vi "axis_scan.vi"(4 "Calibration":bool, 5 "Modes":bool, 6 "Parameters":bool, 7 "Parameters in":T1={"Stimulus"={"Type"=enum."Off", "Phase"=0.0, "Amplitude"=[], "Injection point"=enum."Total pose", "Closed loop"=FALSE, "Offset"=[], "Tip -> world"=FALSE, "Frequency"=0.0, "Length"=0.0}, "Goal Filter A"={"Speedup max"=0.0, "Speedup thresh"=0.0, "Speedup nonlin"=0.0, "Filters"=[]}, "Mode controls"={"Hold"=FALSE, "Cancellation"=FALSE, "Goal filter"=FALSE, "Trigger"=FALSE}, "Manipulator type"=enum."Current piezo", "Manipulator calibration"={"Tool offsets"=[], "Tip light calibration"=[], "Handle light calibration"=[], "Base pivots"=[], "Output pivots"=[], "Length center"=0.0, "Workspace height"=[], "Workspace diameter"=[0.0, 0.0, 36200.0], "Linearization"=[], "Stack travel"=400.0, "Saturation pos"=375.0, "Inverse filters"=[]}, "Network"={"Remote Host"="", "Send Status"=FALSE, "Send Port"=0, "Recv Commands"=FALSE, "Recv Port"=0}, "Goal Filter B"={"Speedup max"=0.0, "Speedup thresh"=0.0, "Speedup nonlin"=0.0, "Filters"=[]}, "Cancellation"={"KP"={"XY"=0.0, "Rxy"=0.0, "Z"=0.0, "Rz"=0.0}, "KI"=0.0, "KD"={"XY"=0.0, "Rxy"=0.0, "Z"=0.0, "Rz"=0.0}, "Max vel"=20.0, "Max acc"=0.001, "Int error limit"=3.0, "RCM gain"=0.0, "Bypass"=FALSE, "Degraded gain"=0.0}, "Transition time"=0.0, "Estimation"={"Link"={"Measure noise"=[], "Process noise"=[], "Alt process noise"=[], "Alt turnoff cycles"=20, "Innovation limit"=[], "Residue threshold"=0.0, "Enable"=FALSE}, "Handle"={"Measure noise"=[], "Process noise"=[], "State limits"=[], "Innovation limit"=[], "Prediction Lookahead"=0.0, "Enable"=FALSE}}} {"Transition time" format="%_3f"; "Cancellation"."Degraded gain" min=0 max=1 step=0.1 format="%#_3p"; "Cancellation"."RCM gain" min=0 max=1 step=0.1 format="%#_3p"; "Cancellation"."KD"."Rz" min=0 max=1 step=0.1 format="%#_3p"; "Cancellation"."KD"."Rxy" min=0 max=1 step=0.1 format="%#_3p"; "Cancellation"."KD"."Z" min=0 max=1 step=0.1 format="%#_3p"; "Cancellation"."KD"."XY" min=0 max=1 step=0.1 format="%#_3p"; "Cancellation"."KI" min=0 max=1 step=0.01 format="%#_3p"; "Cancellation"."KP"."Rz" min=0 max=1 step=0.1 format="%#_3p"; "Cancellation"."KP"."Rxy" min=0 max=1 step=0.1 format="%#_3p"; "Cancellation"."KP"."Z" min=0 max=1 step=0.1 format="%#_3p"; "Cancellation"."KP"."XY" min=0 max=1 step=0.1 format="%#_3p"; "Cancellation"."Max acc" format="%#_3p"; "Goal Filter B"."Filters"."V limit range" format="%_3p"; "Goal Filter B"."Filters"."V limit" format="%_3p"; "Goal Filter B"."Filters"."Upper Q" format="%_3f"; "Goal Filter B"."Filters"."Upper Fc" format="%_3p"; "Goal Filter B"."Filters"."Lower Q" format="%_3f"; "Goal Filter B"."Filters"."Scale factor" format="%_3f"; "Goal Filter B"."Filters"."Lower Fc" format="%_3p"; "Goal Filter B"."Speedup nonlin" format="%_3p"; "Goal Filter B"."Speedup thresh" format="%_3p"; "Goal Filter B"."Speedup max" format="%_3p"; "Manipulator calibration"."Saturation pos" format="%#.1f"; "Manipulator calibration"."Stack travel" format="%#.1f"; "Manipulator calibration"."Output pivots" format="%#_6f"; "Manipulator calibration"."Base pivots" format="%#_6f"; "Manipulator calibration"."Handle light calibration" format="%#.1f"; "Manipulator calibration"."Tip light calibration" format="%#.1f"; "Goal Filter A"."Filters"."V limit range" format="%_3p"; "Goal Filter A"."Filters"."V limit" format="%_3p"; "Goal Filter A"."Filters"."Upper Q" format="%_3f"; "Goal Filter A"."Filters"."Upper Fc" format="%_3p"; "Goal Filter A"."Filters"."Lower Q" format="%_3f"; "Goal Filter A"."Filters"."Scale factor" format="%_3f"; "Goal Filter A"."Filters"."Lower Fc" format="%_3p"; "Goal Filter A"."Speedup nonlin" format="%_3p"; "Goal Filter A"."Speedup thresh" format="%_3p"; "Goal Filter A"."Speedup max" format="%_3p"; "Stimulus"."Length" min=0.0 max=100.0 step=100.0 format="%#_4p"; "Stimulus"."Frequency" min=0.0 step=100.0 format="%#_4g"; "Stimulus"."Offset" format="%#_3p"; "Stimulus"."Amplitude" format="%#_3p"; "Stimulus"."Phase" min=-180.0 max=360.0 step=100.0 format="%#.2f"}, 8 "Next scan occurrence":refnum<k4>, 9 "Use Output Enable":bool, 10 "Amplitude":sgl, 11 "Scan axes":bool[](array[boolean])=[FALSE, FALSE, FALSE, FALSE, FALSE, FALSE]) -> (3 "Got all":bool)   [LabVIEW 2013]
uses:
  testing/Micron params.ctl
  testing/stimulus.ctl
  testing/injection_point.ctl
  filtering/goal_loop_parms.ctl
  testing/mode_conrols.ctl
  testing/manipulator_cal.ctl
  asap/labview/testing/probe_calibration.ctl
  host/network_params.ctl
  cancellation/sq_control_params.ctl
  cancellation/decoupled_gain.ctl
  cancellation/estimation_controls.ctl
  initialization/micron_globals.vi
panel:
  # "Sequence a scan across axes by altering the stimulus amplitude.  If the injection point is in link-length coordinates and \"Use Output Enable\" is true, we also use \"output_enable\" to shut off the other axes.  \n\nThis VI does not return until the entire scan is done.  After starting each trace cycle, we wait for \"Next scan occurrence\" before going on to the next.  This occurrence should be set by the caller when they are done processing the results.  Calls ui_override to control Micron triggering and stimulus.  Additional overrides can be specified by the boolean flags, as for ui_override.   If override is not successful, then we do nothing, and \"Got all\" is false.  Information on the axis currently being driven in stored in the \"Axis scan\" global."
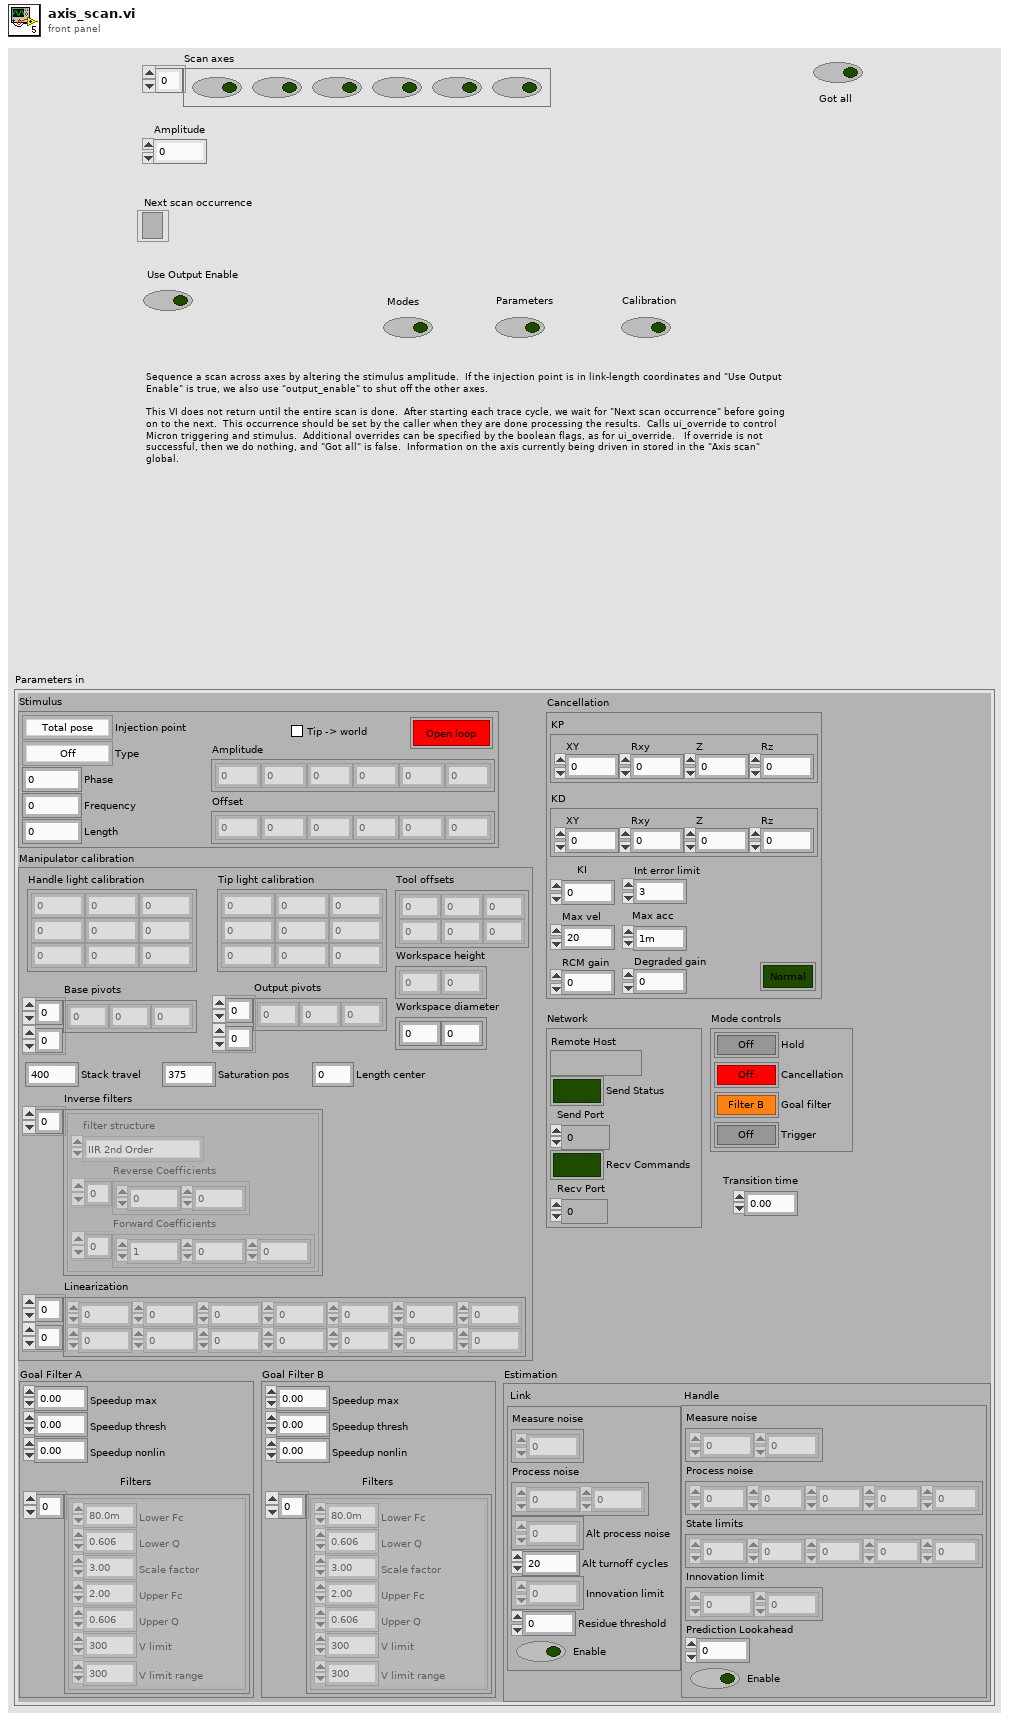
[diagram p1: front panel]
types:
  T1 = typedef "Micron params.ctl" = cluster{"Stimulus":T2, "Goal Filter A":T4, "Mode controls":T5, "Manipulator type":enum16{"Current piezo", "Voltage piezo"}, "Manipulator calibration":T6, "Network":T8, "Goal Filter B":T4, "Cancellation":T9, "Transition time":sgl, "Estimation":T11}
  T2 = typedef "stimulus.ctl" = cluster{"Type":enum16{"Off", "Step", "Sine", "Triangle", "Arbitrary"}, "Phase":dbl, "Amplitude":sgl[], "Injection point":T3, "Closed loop":bool, "Offset":sgl[], "Tip -> world":bool, "Frequency":dbl, "Length":dbl}
  T3 = typedef "injection_point.ctl" = enum16{"Total pose", "V limiter", "Goal ", "Link position", "KF link position", "Inverse kin", "Link goal", "Link error", "Controller", "Output", "Drive", "Light"}
  T4 = typedef "goal_loop_parms.ctl" = cluster{"Speedup max":sgl, "Speedup thresh":sgl, "Speedup nonlin":sgl, "Filters":cluster{"Lower Fc":sgl, "Lower Q":sgl, "Scale factor":sgl, "Upper Fc":sgl, "Upper Q":sgl, "V limit":sgl, "V limit range":sgl}[]}
  T5 = typedef "mode_conrols.ctl" = cluster{"Hold":bool, "Cancellation":bool, "Goal filter":bool, "Trigger":bool}
  T6 = typedef "manipulator_cal.ctl" = cluster{"Tool offsets":sgl[][], "Tip light calibration":T7, "Handle light calibration":T7, "Base pivots":sgl[][], "Output pivots":sgl[][], "Length center":sgl, "Workspace height":sgl[], "Workspace diameter":sgl[], "Linearization":sgl[][], "Stack travel":sgl, "Saturation pos":sgl, "Inverse filters":cluster{"filter structure":enum32{"IIR 2nd Order", "IIR 4th Order"}, "Reverse Coefficients":dbl[], "Forward Coefficients":dbl[]}[]}
  T7 = typedef "probe_calibration.ctl" = sgl[][]
  T8 = typedef "network_params.ctl" = cluster{"Remote Host":string, "Send Status":bool, "Send Port":u16, "Recv Commands":bool, "Recv Port":u16}
  T9 = typedef "sq_control_params.ctl" = cluster{"KP":T10, "KI":sgl, "KD":T10, "Max vel":sgl, "Max acc":sgl, "Int error limit":sgl, "RCM gain":sgl, "Bypass":bool, "Degraded gain":sgl}
  T10 = typedef "decoupled_gain.ctl" = cluster{"XY":sgl, "Rxy":sgl, "Z":sgl, "Rz":sgl}
  T11 = typedef "estimation_controls.ctl" = cluster{"Link":cluster{"Measure noise":dbl[], "Process noise":dbl[], "Alt process noise":dbl[], "Alt turnoff cycles":i32, "Innovation limit":dbl[], "Residue threshold":dbl, "Enable":bool}, "Handle":cluster{"Measure noise":dbl[], "Process noise":dbl[], "State limits":dbl[], "Innovation limit":dbl[], "Prediction Lookahead":sgl, "Enable":bool}}
  T12 = typedef "ui_override_opts.ctl" = cluster{"Triggering":bool, "Parameters":bool, "Stimulus":bool, "Calibration":bool, "Modes":bool}
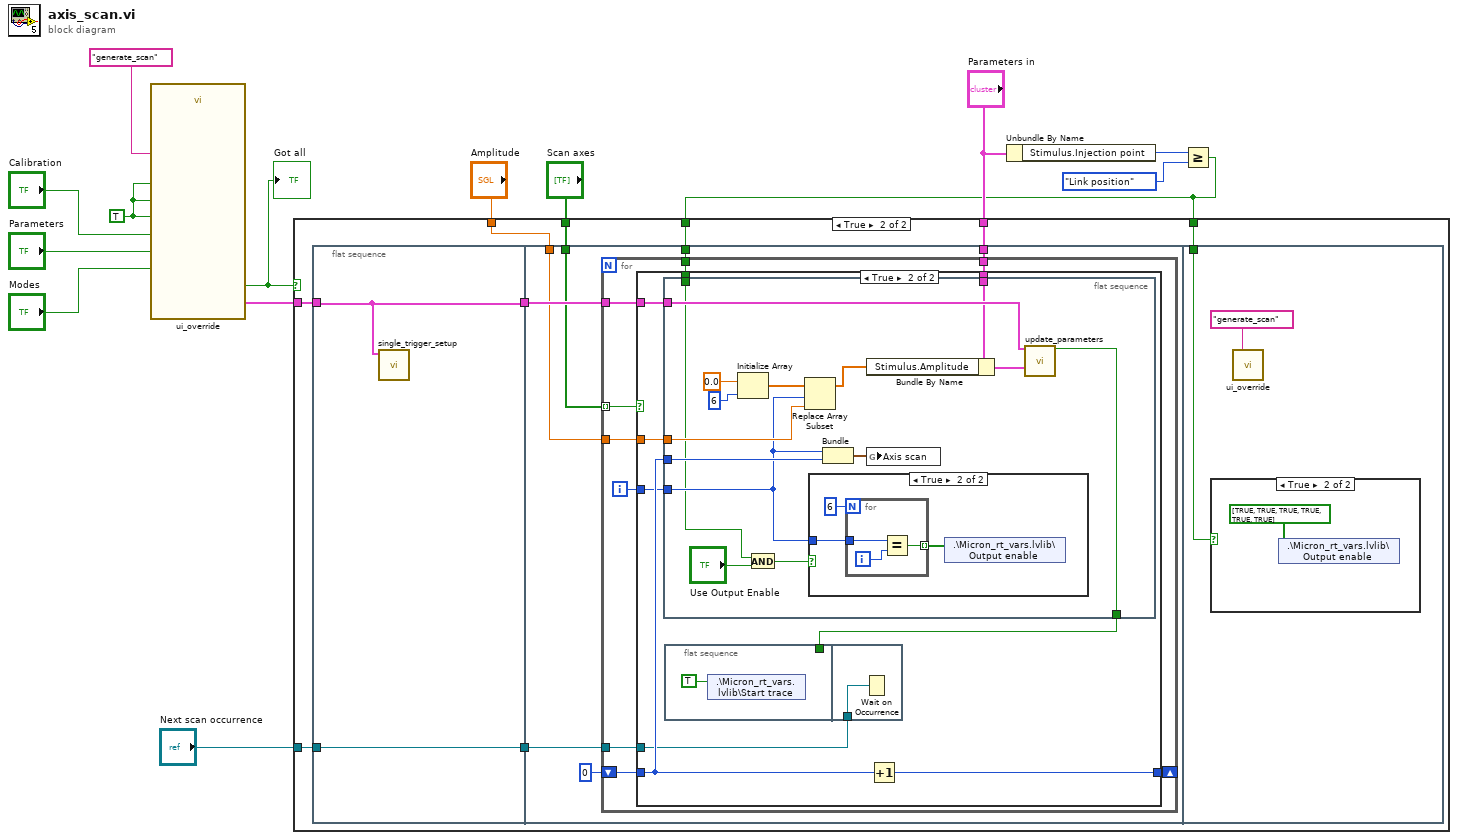
[diagram p0: block diagram]
diagram:
  w10 = TRUE ("Triggering")
  n1 = call "ui_override.vi"("Triggering"=w10, "VI name"="generate_scan", "Parameters"="Parameters", "Stimulus"=w10, "Calibration"="Calibration", "All or nothing"=w10, "Modes"="Modes") -> ("Override"=w12:T12, "Got all"=w11:bool)  [unwired: 6 in, 1 out]
  "Got all" <- w11
  n2 = Unbundle By Name("Parameters in") -> ("Stimulus.Injection point"=w3:T3)
  n3 = Greater Or Equal?(x=w3, y=injection_point."Link position") -> (x >= y?=w1:bool)
  n4 = case shown="True" w11 {
    tunnel: "Next scan occurrence" -> [_ w23]
    tunnel: w12 -> [_ w22]
    tunnel: "Parameters in" -> [_ w19]
    tunnel: "Scan axes" -> [_ w18]
    tunnel: "Amplitude" -> [_ w17]
    tunnel: w1 -> [_ w16]
    tunnel: w1 -> [_ w15]
    frame False {
    }
    frame True {
      n5 = flat-sequence {
        tunnel: w23 -> [w24]
        tunnel: [w24] -> w21
        tunnel: w22 -> [w25]
        tunnel: [w25] -> w20
        tunnel: w21 -> [w31]
        tunnel: w20 -> [w30]
        tunnel: w19 -> [w29]
        tunnel: w18 -> [w28]
        tunnel: w17 -> [w27]
        tunnel: w16 -> [w26]
        tunnel: w15 -> [w75]
        frame #0 {
          n6 = call "single_trigger_setup.vi"("Override in"=w25) -> ()  [unwired: 10 in, 1 out]
        }
        frame #1 {
          n7 = for {
            tunnel: w28 -> [w41] mode=indexing
            shift-right: [w39] -> _
            shift-left: 0 ("dimension size") -> [w40]
            tunnel: w31 -> [w38]
            tunnel: w30 -> [w36]
            tunnel: w29 -> [w35]
            tunnel: w27 -> [w34]
            tunnel: w26 -> [w33]
            i -> [w37]
            n8 = case shown="True" w41 {
              tunnel: w40 -> [w42 w50]
              tunnel: [w42 w51] -> w39
              tunnel: w38 -> [_ w48]
              tunnel: w37 -> [_ w47]
              tunnel: w36 -> [_ w46]
              tunnel: w35 -> [_ w45]
              tunnel: w34 -> [_ w44]
              tunnel: w33 -> [_ w43]
              frame False {
              }
              frame True {
                n9 = flat-sequence {
                  tunnel: w50 -> [w58]
                  tunnel: [w64] -> w49
                  tunnel: w47 -> [w57]
                  tunnel: w46 -> [w63]
                  tunnel: w45 -> [w61]
                  tunnel: w44 -> [w60]
                  tunnel: w43 -> [w55]
                  frame #0 {
                    n10 = Initialize Array(sgl 0.0 ("Amplitude"), 6 ("dimension size")) -> (w66:sgl[])
                    n11 = And(x=w55, y="Use Output Enable") -> (x .and. y?=w54:bool)
                    n12 = Replace Array Subset(array=w66, new element=w60, index=w57) -> (w65:sgl[])
                    n13 = case shown="True" w54 {
                      tunnel: w57 -> [_ w70]
                      frame False {
                      }
                      frame True {
                        n14 = for {
                          N: 6 -> [_]
                          tunnel: w70 -> [w73]
                          tunnel: [w72] -> w69 mode=indexing
                          i -> [w74]
                          n15 = Equal?(x=w73, y=w74) -> (x = y?=w72:bool)
                        }
                        n16 = shared-variable ".\\Micron_rt_vars.lvlib\\Output enable"(w69) -> ()  [unwired: 1 in, 1 out]
                      }
                    }
                    n17 = Bundle(w57, "dimension size"=w58) -> (w59:cluster{i32, "dimension size":i32})  [unwired: 1 in]
                    n18 = Bundle By Name(cluster=w61, "Stimulus.Amplitude"=w65) -> (w62:T1)
                    n19 = global write "micron_globals.vi" "Axis scan"(w59) -> ()
                    n20 = call "update_parameters.vi"("Modify"=w63, "Parameters"=w62) -> ("Changed"=w64:bool)  [unwired: 12 in, 1 out]
                  }
                }
                n21 = flat-sequence {
                  tunnel: w49 -> [_]
                  tunnel: w48 -> [w53]
                  frame #0 {
                    n22 = shared-variable ".\\Micron_rt_vars.lvlib\\Start trace"(TRUE ("Start trace")) -> ()  [unwired: 2 out]
                  }
                  frame #1 {
                    n23 = Wait on Occurrence(2:w53) -> ()  [unwired: 2 in, 1 out]
                  }
                }
                n24 = Increment(x=w50) -> (x+1=w51:i32)
              }
            }
          }
        }
        frame #2 {
          n25 = case shown="True" w75 {
            frame False {
            }
            frame True {
              n26 = shared-variable ".\\Micron_rt_vars.lvlib\\Output enable"(bool[] [TRUE, TRUE, TRUE, TRUE, TRUE, TRUE] ("Output enable")) -> ()  [unwired: 1 in, 1 out]
            }
          }
          n27 = call "ui_override.vi"("VI name"="generate_scan") -> ()  [unwired: 12 in, 3 out]
        }
      }
    }
  }
